vi "Handle Tree Menu Activation.vi"(8 "error in":errorcluster, 9 "Coords":T1, 10 "Menu in":refnum<k9>, 11 "Configuration In":T2) -> (0 "error out":errorcluster, 3 "Discard?":bool)   [LabVIEW 2013, in "LVTM.lvlib"]
uses:
  LVTM.lvlib
  Controls_LVTM/LVTM_Config_Info.ctl
  Controls_LVTM/View.ctl
  Controls_LVTM/SharedDataDVR.ctl
  <vilib>/Utility/miscctls.llb/LVPoint32TypeDef.ctl
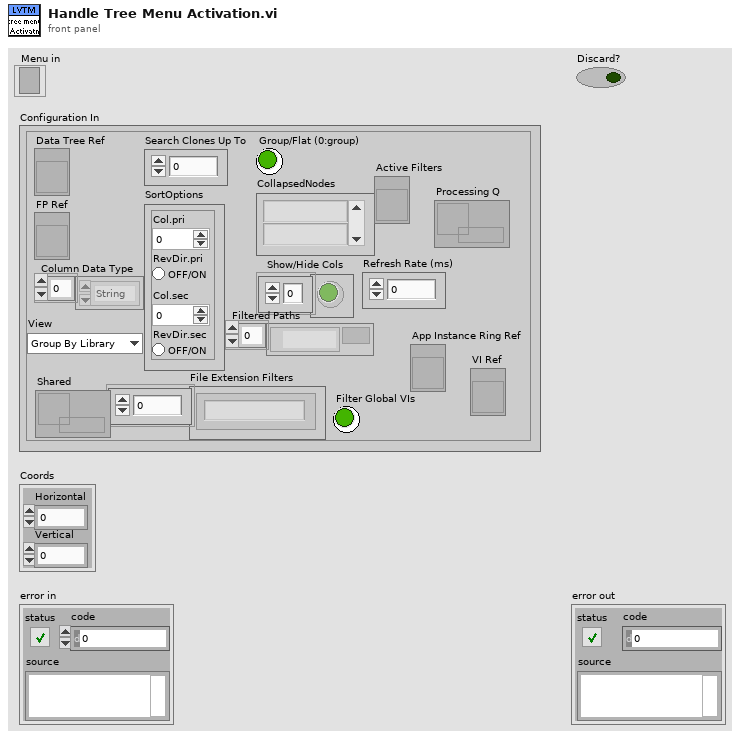
[diagram p1: front panel]
types:
  T1 = typedef "LVPoint32TypeDef.ctl" = cluster{"Horizontal":i32, "Vertical":i32}
  T2 = typedef "LVTM.lvlib/LVTM_Config_Info.ctl" = cluster{"Data Tree Ref":refnum<vi>, "FP Ref":refnum<vi>, "Column Data Type":enum16{"String", "Numeric"}[], "Search Clones Up To":i32, "SortOptions":cluster{"Col.pri":i32, "RevDir.pri":bool, "Col.sec":i32, "RevDir.sec":bool}, "Group/Flat (0:group)":bool, "CollapsedNodes":string[], "Show/Hide Cols":bool[], "Filtered Paths":path[], "View":T3, "File Extension Filters":string[], "Filter Global VIs":bool, "Shared":refnum<data-value>, "Active Filters":refnum<vi>, "Refresh Rate (ms)":i32, "App Instance Ring Ref":refnum<vi>, "Processing Q":refnum<queue>, "VI Ref":refnum<vi>}
  T3 = typedef "LVTM.lvlib/View.ctl" = enum16{"Group By Library", "Group By Folder", "Flat List"}
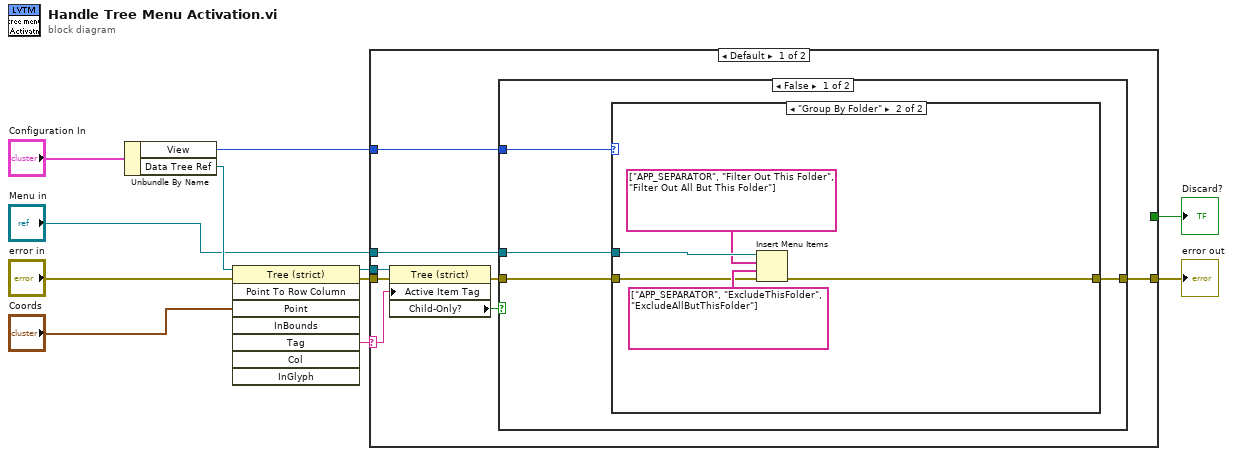
[diagram p0: block diagram]
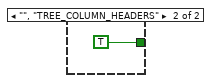
[diagram p4: hidden frame]
diagram:
  n1 = Unbundle By Name("Configuration In") -> ("View"=w1:T3, "Data Tree Ref"=w11:refnum<vi>)
  n2 = invoke class="Tree (strict)" method="Point To Row Column"(reference=w11, error in="error in", "Point"="Coords") -> (reference out=w4:refnum<vi>, error out=w5:errorcluster, "Tag"=w8:string)  [unwired: 5 in, 5 out]
  n3 = case shown="Default" w8 {
    selector: w8 -> [w13 _]
    tunnel: "Menu in" -> [w19 _]
    tunnel: w4 -> [w18 _]
    tunnel: w5 -> [w17 _]
    tunnel: [w14 _] -> w7
    tunnel: [_ TRUE ("Discard?")] -> w9
    tunnel: w1 -> [w12 _]
    frame Default {
      n4 = property class="Tree (strict)"(reference=w18, error in=w17, "Active Item Tag"=w13) -> (error out=w15:errorcluster, "Child-Only?"=w16:bool)  [unwired: 1 out]
      n5 = case shown="False" w16 {
        tunnel: w19 -> [w23 _]
        tunnel: w15 -> [w22 w30]
        tunnel: [w21 w30] -> w14
        tunnel: w12 -> [w20 _]
        frame False {
          n6 = case shown="\"Group By Folder\"" w20 {
            tunnel: w23 -> [_ w29]
            tunnel: w22 -> [w24 w26]
            tunnel: [w24 w25] -> w21
            frame "Group By Library", Default {
            }
            frame "Group By Folder" {
              n7 = Insert Menu Items(6:w26, 7:string[] ["APP_SEPARATOR", "ExcludeThisFolder", "ExcludeAllButThisFolder"] ("item tags"), 8:string[] ["APP_SEPARATOR", "Filter Out This Folder", "Filter Out All But This Folder"] ("item names"), 9:w29) -> (0:w25:errorcluster)  [unwired: 2 in, 2 out]
            }
          }
        }
        frame True {
        }
      }
    }
    frame "", "TREE_COLUMN_HEADERS" {
    }
  }
  "Discard?" <- w9
  "error out" <- w7
